vi "Tank Data Global.vi"(7 "Pump Data Mode":T1, 8 "Cal Coefficients":dbl[][](array[numeric]), 11 "Tank Data IN":dbl[](array[numeric])) -> (3 "Tank Data OUT":dbl[](array[numeric]))   [LabVIEW 2013]
uses:
  Type Defs/Pump Data Mode.ctl
  <vilib>/ptbypt/NI_PtbyPt.lvlib
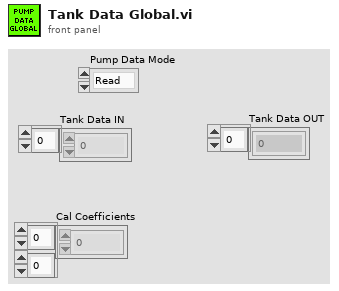
[diagram p1: front panel]
types:
  T1 = typedef "Pump Data Mode.ctl" = enum16{"Read", "Write Data", "Write Cal"}
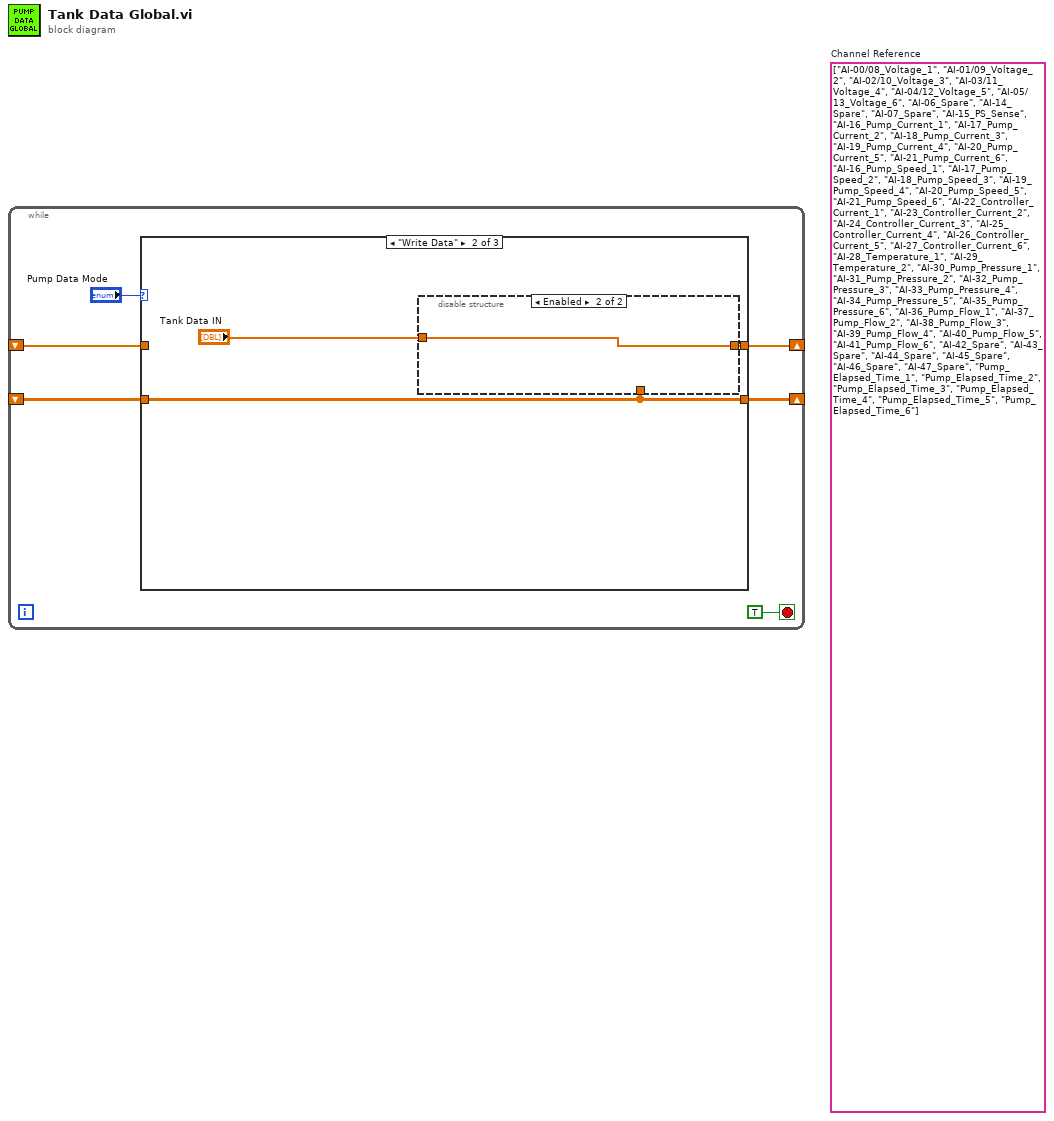
[diagram p0: block diagram]
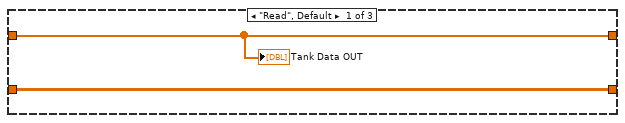
[diagram p2: hidden frame]
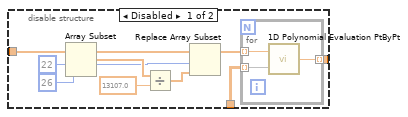
[diagram p3: hidden frame]
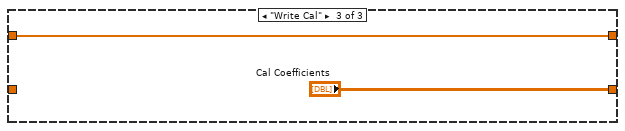
[diagram p4: hidden frame]
diagram:
  (unwired) string[] ["AI-00/08_Voltage_1", "AI-01/09_Voltage_2", "AI-02/10_Voltage_3", "AI-03/11_Voltage_4", "AI-04/12_Voltage_5", "AI-05/13_Voltage_6", "AI-06_Spare", "AI-14_Spare", "AI-07_Spare", "AI-15_PS_Sense", "AI-16_Pump_Current_1", "AI-17_Pump_Current_2", "AI-18_Pump_Current_3", "AI-19_Pump_Current_4", "AI-20_Pump_Current_5", "AI-21_Pump_Current_6", "AI-16_Pump_Speed_1", "AI-17_Pump_Speed_2", "AI-18_Pump_Speed_3", "AI-19_Pump_Speed_4", "AI-20_Pump_Speed_5", "AI-21_Pump_Speed_6", "AI-22_Controller_Current_1", "AI-23_Controller_Current_2", "AI-24_Controller_Current_3", "AI-25_Controller_Current_4", "AI-26_Controller_Current_5", "AI-27_Controller_Current_6", "AI-28_Temperature_1", "AI-29_Temperature_2", "AI-30_Pump_Pressure_1", "AI-31_Pump_Pressure_2", "AI-32_Pump_Pressure_3", "AI-33_Pump_Pressure_4", "AI-34_Pump_Pressure_5", "AI-35_Pump_Pressure_6", "AI-36_Pump_Flow_1", "AI-37_Pump_Flow_2", "AI-38_Pump_Flow_3", "AI-39_Pump_Flow_4", "AI-40_Pump_Flow_5", "AI-41_Pump_Flow_6", "AI-42_Spare", "AI-43_Spare", "AI-44_Spare", "AI-45_Spare", "AI-46_Spare", "AI-47_Spare", "Pump_Elapsed_Time_1", "Pump_Elapsed_Time_2", "Pump_Elapsed_Time_3", "Pump_Elapsed_Time_4", "Pump_Elapsed_Time_5", "Pump_Elapsed_Time_6"]  # Channel Reference
  n1 = while {
    shift-right: [w5] -> _
    shift-left: _ -> [w4]
    shift-right: [w2] -> _
    shift-left: _ -> [w1]
    stop <- TRUE stop-if-true
    n2 = case shown="\"Write Data\"" "Pump Data Mode" {
      tunnel: [w8 w11 w25] -> w5
      tunnel: w4 -> [w8 _ w25]
      tunnel: [w7 w10 "Cal Coefficients"] -> w2
      tunnel: w1 -> [w7 w10 _]
      frame "Read", Default {
        "Tank Data OUT" <- w8
      }
      frame "Write Data" {
        n3 = disable-structure shown="Enabled" {
          disable-tunnel: [w20 w24] -> w11
          disable-tunnel: w10 -> [w19 _]
          disable-tunnel: "Tank Data IN" -> [w12 w24]
          frame Disabled {
            w14 = 22 ("index")
            n4 = Array Subset(array=w12, index=w14, length=26) -> (w15:dbl[])
            n5 = Divide(x=w15, y=13107.0) -> (x/y=w17:dbl[])
            n6 = Replace Array Subset(array=w12, new element=w17, index=w14) -> (w18:dbl[])
            n7 = for {
              tunnel: w19 -> [w23] mode=indexing
              tunnel: w18 -> [w22] mode=indexing
              tunnel: [w21] -> w20 mode=indexing
              n8 = call <vilib>:"1D Polynomial Evaluation PtByPt.vi"("Coefficients: a"=w23, "x"=w22) -> ("y"=w21:dbl)
            }
          }
          frame Enabled {
          }
        }
      }
      frame "Write Cal" {
      }
    }
  }
